vi "makeResult.vi"(8 "error in (no error)":errorcluster, 11 "TextTestRunner in":refnum<class "TextTestRunner.lvclass">) -> (0 "error out":errorcluster, 2 "TestResult":refnum<class "TestResult.lvclass">, 3 "TextTestRunner out":refnum<class "TextTestRunner.lvclass">)   [LabVIEW 2013, in "TextTestRunner.lvclass"]
uses:
  TextTestRunner.lvclass
  TestResult/TestResult.lvclass
  TextTestRunner.lvclass/TextTestRunner.ctl
  _TextTestResult/_TextTestResult.lvclass
panel:
  # "JKI VI Tester for LabVIEW\nhttp://jkisoft.com/vi-tester\nCopyright (C) 2007-2009, JKI <info@jkisoft.com>\nALL RIGHTS RESERVED"
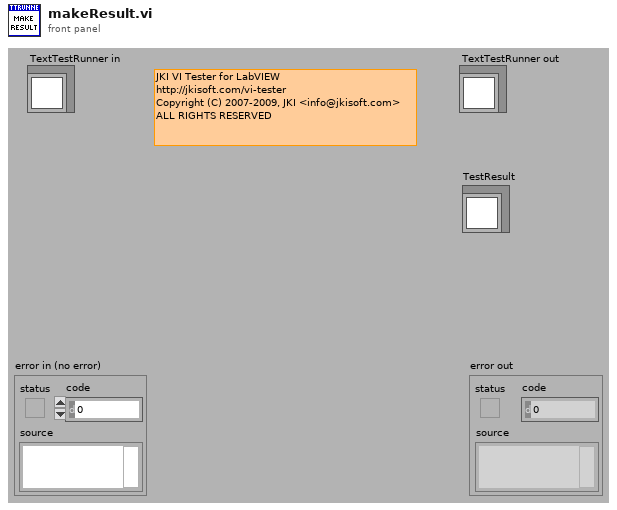
[diagram p1: front panel]
types:
  T1 = typedef "TestRunner.lvclass/PublicEvents--Cluster.ctl" = cluster{"abortEventRef":refnum<user-event>, "resultStatusChangedEventRef":refnum<user-event>, "testStartedEventRef":refnum<user-event>}
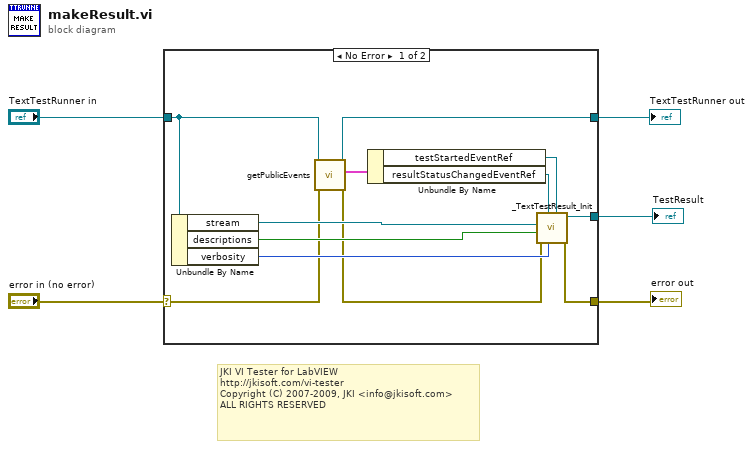
[diagram p0: block diagram]
diagram:
  # "JKI VI Tester for LabVIEW\nhttp://jkisoft.com/vi-tester\nCopyright (C) 2007-2009, JKI <info@jkisoft.com>\nALL RIGHTS RESERVED"
  n1 = case shown="No Error" "error in (no error)" {
    selector: "error in (no error)" -> [w8 w19]
    tunnel: [w14 w19] -> w4
    tunnel: [w11 w18] -> w2
    tunnel: "TextTestRunner in" -> [w12 w18]
    tunnel: [w13 _] -> w1
    frame No Error {
      n2 = Unbundle By Name(w12) -> ("stream"=w17:refnum<queue>, "descriptions"=w16:bool, "verbosity"=w15:u32)
      n3 = call-dynamic "getPublicEvents.vi"("error in (no error)"=w8, "TextTestRunner in"=w12) -> ("error out"=w7:errorcluster, "publicEvents"=w10:T1, "TextTestRunner out"=w11:refnum<class "TextTestRunner.lvclass">)  [unwired: 7 in]
      n4 = Unbundle By Name(w10) -> ("testStartedEventRef"=w6:refnum<user-event>, "resultStatusChangedEventRef"=w9:refnum<user-event>)
      n5 = call "_TextTestResult_Init.vi"("testStartedEventRef"=w6, "verbosity"=w15, "resultStatusChangedEventRef"=w9, "error in (no error)"=w7, "descriptions"=w16, "stream"=w17) -> ("error out"=w14:errorcluster, "TestTestResult out"=w13:refnum<class "_TextTestResult.lvclass">)  [unwired: 4 in]
    }
    frame Error {
    }
  }
  "error out" <- w4
  "TextTestRunner out" <- w2
  "TestResult" <- w1
